vi "Continuous Acquisition to File.vi"() -> ()   [LabVIEW 2020]
uses:
  <vilib>/DAQmx/read.llb/DAQmx Read (Analog 2D DBL NChan NSamp).vi
  <vilib>/DAQmx/create/channels.llb/DAQmx Create Channel (AI-Voltage-Basic).vi
  <vilib>/DAQmx/configure/timing.llb/DAQmx Timing (Sample Clock).vi
  <vilib>/DAQmx/miscellaneous.llb/DAQmx Fill In Error Info.vi
  <resource>/objmgr/daqmx.rc
panel:
  in  "Minimum sample to read":i32
  in  "Path":path
  out "Waveform Chart":dbl[][](graph)
  in  "stop":bool
  out "Samples in Buffer":i32
  out "Boolean":bool
  in  "Buffer Read Rate":u32
  in  "Buffer size (sample per channel)":i32=1000
  in  "rate":dbl=1000.0 format="%0.2f"
  in  "DAQmx Physical Channel":tag
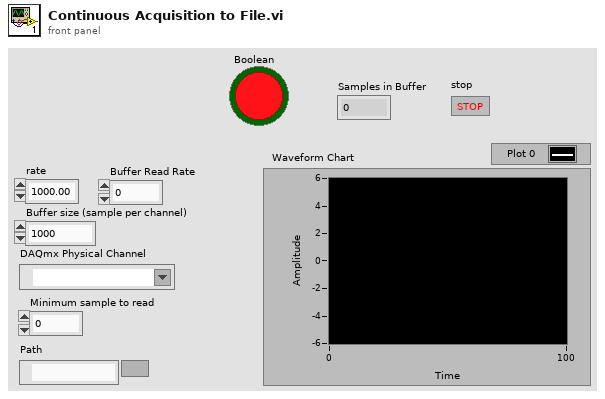
[diagram p1: front panel]
types:
  T1 = enum16{"open", "replace", "create", "open or create", "replace or create", "replace or create with confirmation"}
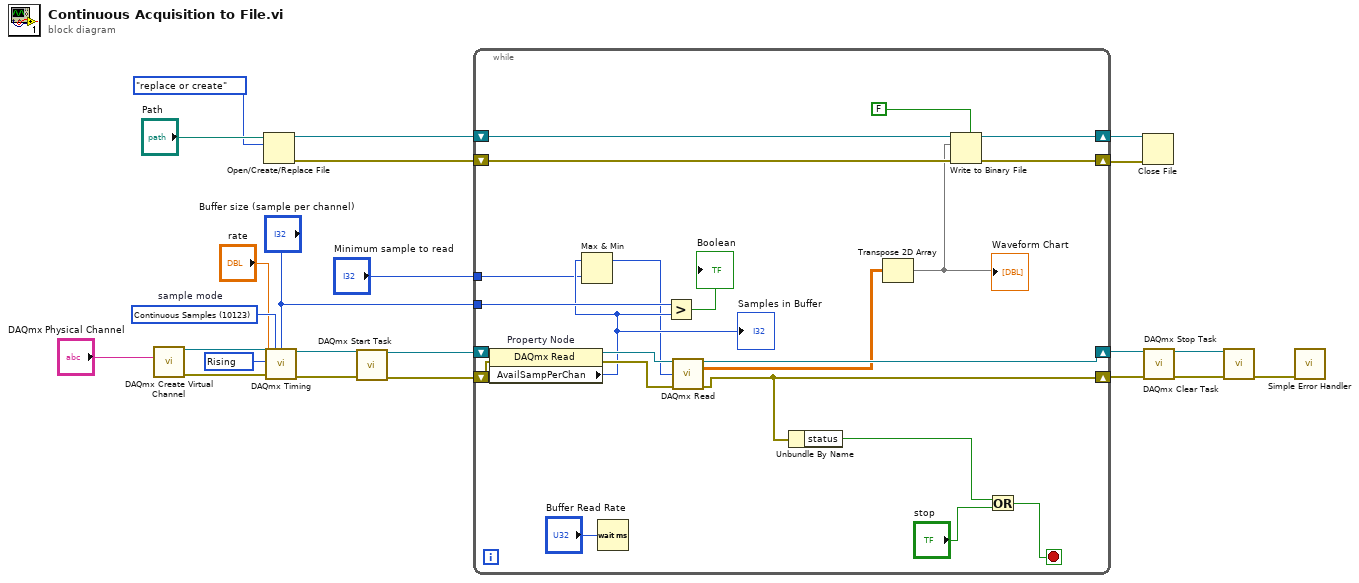
[diagram p0: block diagram]
diagram:
  w9 = 10280 items=["Rising"=10280, "Falling"=10171] ("active edge")
  w20 = 10123 items=["Finite Samples"=10178, "Continuous Samples"=10123, "Hardware Timed Single Point"=12522]  # sample mode
  n1 = call-poly <vilib>:"DAQmx Create Virtual Channel.vi"("physical channels"="DAQmx Physical Channel") -> ("task out"=w22:refnum<k21>, "error out"=w21:errorcluster)  [unwired: 13 in]
  n2 = Open/Create/Replace File(file path (use dialog)="Path", operation (0:open)=T1."replace or create") -> (refnum out=w5:refnum<file>, error out=w4:errorcluster)  [unwired: 4 in, 1 out]
  n3 = call-poly <vilib>:"DAQmx Timing.vi"("task/channels in"=w22, "sample mode"=w20, "samples per channel"="Buffer size (sample per channel)", "rate"="rate", "active edge"=w9, "error in"=w21) -> ("task out"=w18:refnum<k21>, "error out"=w17:errorcluster)  [unwired: 8 in]
  n4 = call <vilib>:"DAQmx Start Task.vi"("task/channels in"=w18, "error in"=w17) -> ("task out"=w16:refnum<k21>, "error out"=w15:errorcluster)  [unwired: 12 in]
  n5 = while {
    tunnel: "Buffer size (sample per channel)" -> [w40]
    shift-right: [w34] -> w13
    shift-left: w16 -> [w45]
    shift-right: [w35] -> w12
    shift-left: w15 -> [w44]
    tunnel: "Minimum sample to read" -> [w27]
    shift-right: [w26] -> w2
    shift-left: w5 -> [w33]
    shift-right: [w25] -> w1
    shift-left: w4 -> [w32]
    stop <- w37 stop-if-true
    n6 = property on="Property Node" class="DAQmx Read"(reference=w45, error in=w44) -> (reference out=w43:refnum<k21>, error out=w42:errorcluster, "AvailSampPerChan"=w31:u32)
    "Samples in Buffer" <- w31
    n7 = Max & Min(x=w31, y=w27) -> (max(x,y)=w30:u32)  [unwired: 1 out]
    n8 = Wait (ms)(milliseconds to wait="Buffer Read Rate") -> ()  [unwired: 1 out]
    n9 = Greater?(x=w40, y=w31) -> (0:→"Boolean":bool)
    n10 = call-poly <vilib>:"DAQmx Read.vi"("task/channels in"=w43, "number of samples per channel"=w30, "error in"=w42) -> ("task out"=w34:refnum<k21>, "data"=w28:dbl[][], "error out"=w35:errorcluster)  [unwired: 10 in]
    n11 = Unbundle By Name(w35) -> ("status"=w38:bool)
    n12 = Transpose 2D Array(2D array=w28) -> (transposed array=w24:dbl[][])
    "Waveform Chart" <- w24
    n13 = Write to Binary File(file (use dialog)=w33, data=w24, error in=w32, 5:FALSE ("prepend array or string size? (T)")) -> (refnum out=w26:refnum<file>, error out=w25:errorcluster)  [unwired: 2 in, 1 out]
    n14 = Or(x=w38, y="stop") -> (x .or. y?=w37:bool)
  }
  n15 = Close File(refnum=w2, error in=w1) -> ()  [unwired: 2 out]
  n16 = call <vilib>:"DAQmx Stop Task.vi"("task/channels in"=w13, "error in"=w12) -> ("task out"=w11:refnum<k21>, "error out"=w10:errorcluster)  [unwired: 12 in]
  n17 = call <vilib>:"DAQmx Clear Task.vi"("task in"=w11, "error in"=w10) -> ("error out"=w8:errorcluster)  [unwired: 13 in]
  n18 = call <vilib>:"Simple Error Handler.vi"("error in (no error)"=w8) -> ()  [unwired: 4 in, 5 out]
